vi "Download File from Internet.vi"(4 "Error In":errorcluster, 6 "Download to (temp folder)":path=path "", 7 "URL to File":string) -> (0 "Error Out":errorcluster, 2 "File Type":string, 3 "Downloaded File":path)   [LabVIEW 2015]
doc: "Downloads file from internet.\nIf \"Download to\" input isn't wired, file is stored in temporary directory.\nIf \"Download to\" is a folder, file is stored there with original file name.\nIf \"Download to\" is a file, file is written to that file name."
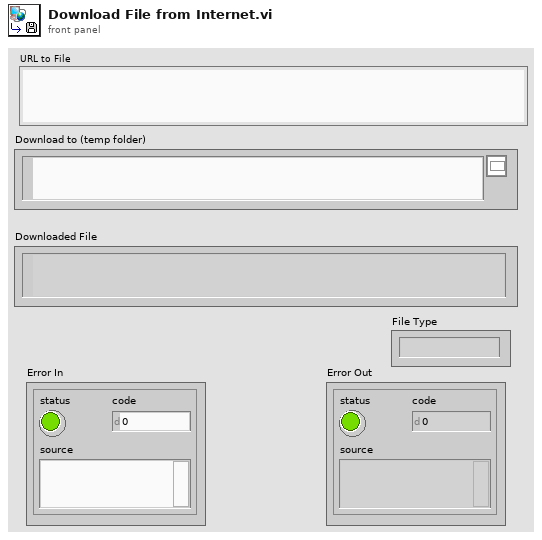
[diagram p1: front panel]
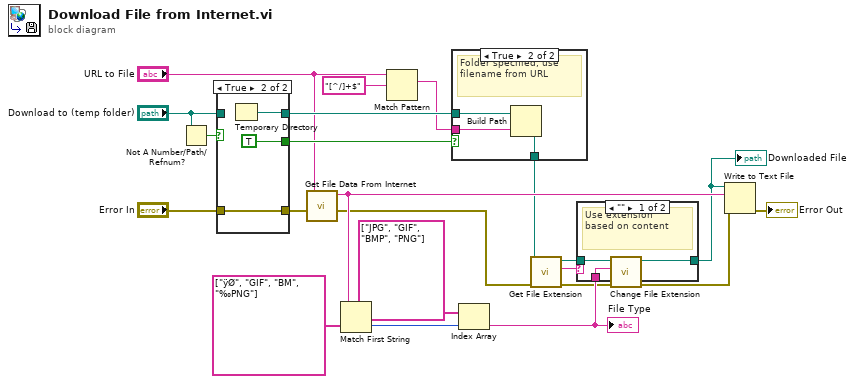
[diagram p0: block diagram]
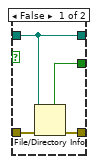
[diagram p3: hidden frame]
diagram:
  n1 = Not A Number/Path/Refnum?(number/path/refnum="Download to (temp folder)") -> (NaN/Path/Refnum?=w15:bool)
  n2 = case shown="True" w15 {
    tunnel: [w25 TRUE ("directory")] -> w20
    tunnel: "Download to (temp folder)" -> [w22 _]
    tunnel: "Error In" -> [w24 w26]
    tunnel: [w23 w26] -> w18
    tunnel: [w22 w28] -> w14
    frame False {
      n3 = File/Directory Info(path=w22, error in=w24) -> (directory=w25:bool, error out=w23:errorcluster)  [unwired: 5 out]
    }
    frame True {
      n4 = Temporary Directory() -> (w28:path)
    }
  }
  n5 = call "Get File Data From Internet.vi"("Error In"=w18, "URL to File"="URL to File") -> ("error out"=w2:errorcluster, "File data"=w8:string)  [unwired: 4 in]
  n6 = Match First String(2:string[] ["ÿØ", "GIF", "BM", "‰PNG"], 3:w8) -> (0:w10:i32)  [unwired: 1 out]
  n7 = Match Pattern(string="URL to File", regular expression="[^/]+$") -> (match substring=w12:string)  [unwired: 1 in, 3 out]
  n8 = case shown="True" w20 {
    tunnel: w14 -> [w29 w32]
    tunnel: w12 -> [_ w31]
    tunnel: [w29 w30] -> w4
    frame False {
      # "Filename specified.\nUse it."
    }
    frame True {
      # "Folder specified, use filename from URL"
      n9 = Build Path(base path=w32, name or relative path=w31) -> (appended path=w30:path)
    }
  }
  n10 = Index Array(array=string[] ["JPG", "GIF", "BMP", "PNG"], index=w10) -> (element=w5:string)
  "File Type" <- w5
  n11 = call <vilib>:"Get File Extension.vi"("error in (no error)"=w2, "file"=w4) -> ("error out"=w1:errorcluster, "lowercase file extension"=w6:string, "dup file"=w7:path)  [unwired: 5 in, 2 out]
  n12 = case shown="\"\"" w6 {
    tunnel: w7 -> [w35 w36]
    tunnel: [w34 w36] -> w3
    tunnel: w5 -> [w33 _]
    frame "" {
      # "Use extension\nbased on content"
      n13 = call "Change File Extension.vi"("New extension"=w33, "File Path In"=w35) -> ("File Path Out"=w34:path)  [unwired: 3 in]
    }
    frame Default {
      # "Use existing\nextension"
    }
  }
  "Downloaded File" <- w3
  n14 = Write to Text File(file (use dialog)=w3, text=w8, error in=w1) -> (error out=→"Error Out":errorcluster)  [unwired: 1 in, 2 out]
